vi "Coffee_Machine.vi"() -> ()   [LabVIEW 2014]
panel:
  in  "stop":bool
  out "Your Drink in Progress":u8(slide) scale=0.0..100.0
  out "Coffee Out?":bool
  out "Water Out?":bool
  out "Tea Out?":bool
  out "Milk Out?":bool
  in  "Tea":bool
  in  "Coffee":bool
  in  "Milk":bool
  out "Water  (ml)":dbl(slide) scale=0.0..10000.0
  out "Tea Powder (gms)":dbl(slide) scale=0.0..10000.0
  out "Coffee Powder (gms)":dbl(slide) scale=0.0..10000.0
  out "Milk (ml)":dbl(slide) scale=0.0..10000.0
  in  "Error In":errorcluster
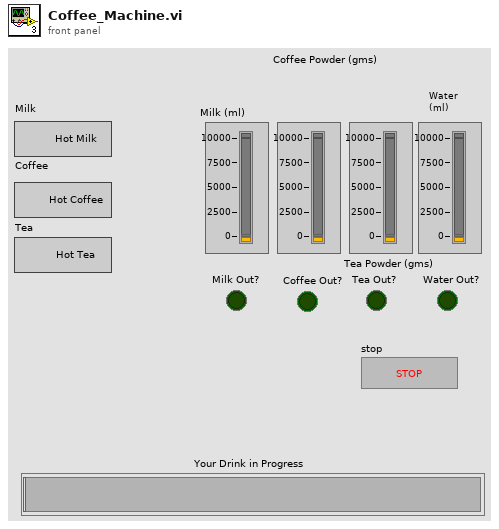
[diagram p1: front panel]
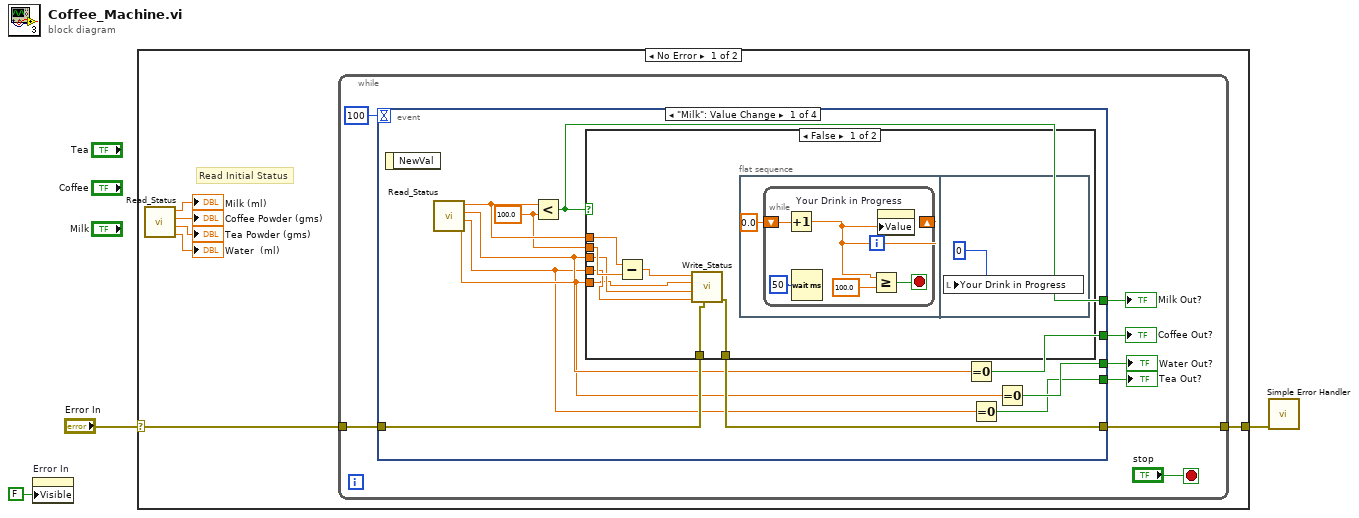
[diagram p0: block diagram]
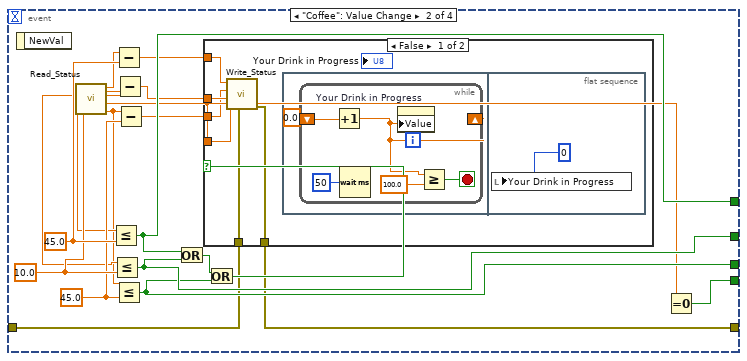
[diagram p3: hidden frame]
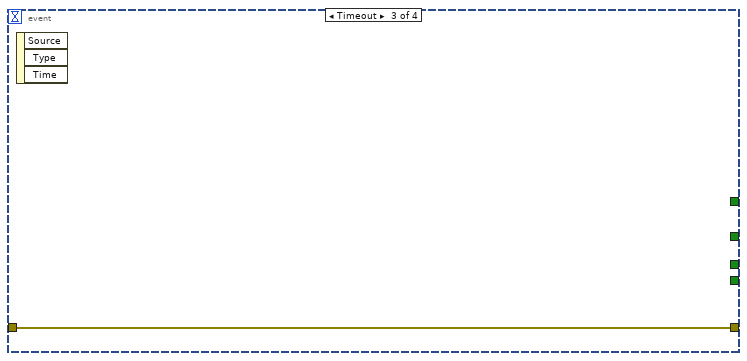
[diagram p5: hidden frame]
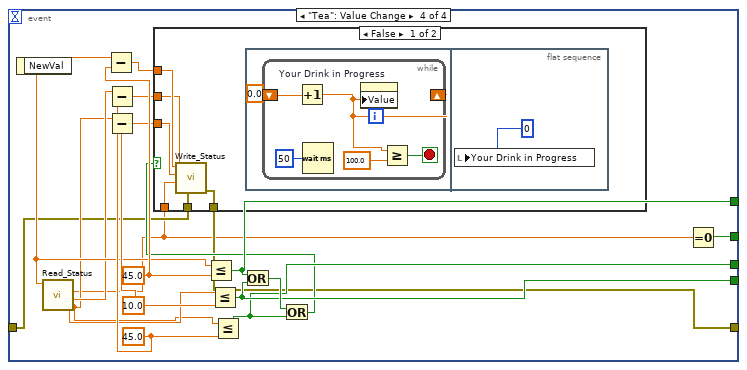
[diagram p6: hidden frame]
diagram:
  n1 = property on="Error In" class="Clust (strict)"("Visible"=FALSE) -> ()  [unwired: 2 in, 2 out]
  n2 = case shown="No Error" "Error In" {
    selector: "Error In" -> [w9 w110]
    tunnel: [w4 w110] -> w2
    frame No Error {
      # "Read Initial Status"
      n3 = call "Read_Status.vi"() -> ("Water\n   (Lt)"=→"Water  (ml)":dbl, "Tea Powder\n       (Kg)"=→"Tea Powder (gms)":dbl, "Coffee Powder\n         (Kg)"=→"Coffee Powder (gms)":dbl, "Milk\n (Lt)"=→"Milk (ml)":dbl)  [unwired: 8 in]
      n4 = while {
        tunnel: w9 -> [w17]
        tunnel: [w11] -> w4
        stop <- "stop" stop-if-true
        n5 = event shown="[0] \"Milk\": Value Change" {
          selector: _ -> [_ _ _ _]
          dyn-events: _ -> [_ _ _ _]
          timeout: 100 -> [_ _ _ _]
          tunnel: w17 -> [w26 w52 w77 w83]
          tunnel: [w18 w61 _ w94] -> w16
          tunnel: [w24 w60 _ w91] -> w15
          tunnel: [w23 w59 _ w92] -> w14
          tunnel: [w22 w55 _ w93] -> w13
          tunnel: [w25 w51 w77 w82] -> w11
          event "Milk": Value Change {
            w27 = 100.0 ("y")
            n6 = event-data() -> ()  [unwired: 1 in, 1 out]
            n7 = call "Read_Status.vi"() -> ("Water\n   (Lt)"=w20:dbl, "Tea Powder\n       (Kg)"=w19:dbl, "Coffee Powder\n         (Kg)"=w21:dbl, "Milk\n (Lt)"=w28:dbl)  [unwired: 8 in]
            n8 = Less?(x=w28, y=w27) -> (x < y?=w18:bool)
            n9 = case shown="False" w18 {
              tunnel: w28 -> [w36 _]
              tunnel: w27 -> [w35 _]
              tunnel: w21 -> [w33 _]
              tunnel: w19 -> [w32 _]
              tunnel: w20 -> [w31 _]
              tunnel: w26 -> [w30 w44]
              tunnel: [w29 w44] -> w25
              frame False {
                n10 = Subtract(x=w36, y=w35) -> (x-y=w34:dbl)
                n11 = call "Write_Status.vi"("Error In"=w30, "Tea Powder\n       (Kg)"=w32, "Coffee Powder\n         (Kg)"=w33, "Water\n   (Lt)"=w31, "Milk\n (Lt)"=w34) -> ("Error Out"=w29:errorcluster)  [unwired: 6 in]
                n12 = flat-sequence {
                  frame #0 {
                    n13 = while {
                      shift-right: [w38] -> _
                      shift-left: 0.0 -> [w41]
                      stop <- w40 stop-if-true
                      n14 = Increment(x=w41) -> (x+1=w38:dbl)
                      n15 = Wait (ms)(milliseconds to wait=u32 50) -> ()  [unwired: 1 out]
                      n16 = Greater Or Equal?(x=w38, y=100.0) -> (x >= y?=w40:bool)
                      n17 = property on="Your Drink in Progress" class="Slide (strict)"("Value"=w38) -> ()  [unwired: 2 in, 2 out]
                    }
                  }
                  frame #1 {
                    n18 = local write "Your Drink in Progress"(u8 0 ("Your Drink in Progress")) -> ()
                  }
                }
              }
              frame True {
              }
            }
            n19 = Equal To 0?(x=w21) -> (x = 0?=w24:bool)
            n20 = Equal To 0?(x=w19) -> (x = 0?=w22:bool)
            n21 = Equal To 0?(x=w20) -> (x = 0?=w23:bool)
          }
          event "Coffee": Value Change {
            w56 = 45.0 ("y")
            w57 = 10.0 ("y")
            w58 = 45.0 ("y")
            n22 = event-data() -> ()  [unwired: 1 in, 1 out]
            n23 = call "Read_Status.vi"() -> ("Water\n   (Lt)"=w47:dbl, "Tea Powder\n       (Kg)"=w45:dbl, "Coffee Powder\n         (Kg)"=w49:dbl, "Milk\n (Lt)"=w53:dbl)  [unwired: 8 in]
            n24 = Less Or Equal?(x=w53, y=w58) -> (x <= y?=w61:bool)
            n25 = Less Or Equal?(x=w49, y=w57) -> (x <= y?=w60:bool)
            n26 = Subtract(x=w53, y=w58) -> (x-y=w50:dbl)
            n27 = Less Or Equal?(x=w47, y=w56) -> (x <= y?=w59:bool)
            n28 = Subtract(x=w49, y=w57) -> (x-y=w48:dbl)
            n29 = Subtract(x=w47, y=w56) -> (x-y=w46:dbl)
            n30 = Or(x=w61, y=w60) -> (x .or. y?=w62:bool)
            n31 = Or(x=w62, y=w59) -> (x .or. y?=w54:bool)
            n32 = case shown="False" w54 {
              tunnel: w52 -> [w68 w76]
              tunnel: [w67 w76] -> w51
              tunnel: w50 -> [w66 _]
              tunnel: w48 -> [w65 _]
              tunnel: w46 -> [w64 _]
              tunnel: w45 -> [w63 _]
              frame False {
                n33 = call "Write_Status.vi"("Error In"=w68, "Tea Powder\n       (Kg)"=w63, "Coffee Powder\n         (Kg)"=w65, "Water\n   (Lt)"=w64, "Milk\n (Lt)"=w66) -> ("Error Out"=w67:errorcluster)  [unwired: 6 in]
                n34 = flat-sequence {
                  frame #0 {
                    n35 = while {
                      shift-right: [w70] -> _
                      shift-left: 0.0 -> [w73]
                      stop <- w72 stop-if-true
                      n36 = Increment(x=w73) -> (x+1=w70:dbl)
                      n37 = Wait (ms)(milliseconds to wait=u32 50) -> ()  [unwired: 1 out]
                      n38 = property on="Your Drink in Progress" class="Slide (strict)"("Value"=w70) -> ()  [unwired: 2 in, 2 out]
                      n39 = Greater Or Equal?(x=w70, y=100.0) -> (x >= y?=w72:bool)
                    }
                  }
                  frame #1 {
                    n40 = local write "Your Drink in Progress"(u8 0 ("Your Drink in Progress")) -> ()
                  }
                }
              }
              frame True {
              }
            }
            n41 = Equal To 0?(x=w45) -> (x = 0?=w55:bool)
          }
          event Timeout {
            n42 = event-data() -> ()  [unwired: 1 in, 3 out]
          }
          event "Tea": Value Change {
            w88 = 45.0 ("y")
            w89 = 10.0 ("y")
            w90 = 45.0 ("y")
            n43 = event-data() -> ()  [unwired: 1 in, 1 out]
            n44 = call "Read_Status.vi"() -> ("Water\n   (Lt)"=w85:dbl, "Tea Powder\n       (Kg)"=w86:dbl, "Coffee Powder\n         (Kg)"=w78:dbl, "Milk\n (Lt)"=w87:dbl)  [unwired: 8 in]
            n45 = Subtract(x=w87, y=w90) -> (x-y=w81:dbl)
            n46 = Subtract(x=w86, y=w89) -> (x-y=w80:dbl)
            n47 = Subtract(x=w85, y=w88) -> (x-y=w79:dbl)
            n48 = Less Or Equal?(x=w87, y=w90) -> (x <= y?=w94:bool)
            n49 = Less Or Equal?(x=w86, y=w89) -> (x <= y?=w93:bool)
            n50 = Less Or Equal?(x=w85, y=w88) -> (x <= y?=w92:bool)
            n51 = Or(x=w94, y=w93) -> (x .or. y?=w95:bool)
            n52 = Or(x=w95, y=w92) -> (x .or. y?=w84:bool)
            n53 = case shown="False" w84 {
              tunnel: w83 -> [w101 w109]
              tunnel: [w100 w109] -> w82
              tunnel: w81 -> [w99 _]
              tunnel: w80 -> [w98 _]
              tunnel: w79 -> [w97 _]
              tunnel: w78 -> [w96 _]
              frame False {
                n54 = call "Write_Status.vi"("Error In"=w101, "Tea Powder\n       (Kg)"=w98, "Coffee Powder\n         (Kg)"=w96, "Water\n   (Lt)"=w97, "Milk\n (Lt)"=w99) -> ("Error Out"=w100:errorcluster)  [unwired: 6 in]
                n55 = flat-sequence {
                  frame #0 {
                    n56 = while {
                      shift-right: [w103] -> _
                      shift-left: 0.0 -> [w106]
                      stop <- w105 stop-if-true
                      n57 = Increment(x=w106) -> (x+1=w103:dbl)
                      n58 = Wait (ms)(milliseconds to wait=u32 50) -> ()  [unwired: 1 out]
                      n59 = property on="Your Drink in Progress" class="Slide (strict)"("Value"=w103) -> ()  [unwired: 2 in, 2 out]
                      n60 = Greater Or Equal?(x=w103, y=100.0) -> (x >= y?=w105:bool)
                    }
                  }
                  frame #1 {
                    n61 = local write "Your Drink in Progress"(u8 0 ("Your Drink in Progress")) -> ()
                  }
                }
              }
              frame True {
              }
            }
            n62 = Equal To 0?(x=w78) -> (x = 0?=w91:bool)
          }
        }
        "Coffee Out?" <- w15
        "Water Out?" <- w14
        "Tea Out?" <- w13
        "Milk Out?" <- w16
      }
    }
    frame Error {
    }
  }
  n63 = call <vilib>:"Simple Error Handler.vi"("error in (no error)"=w2) -> ()  [unwired: 4 in, 5 out]
